vi "startTransport.vi"(8 "error in (no error)":errorcluster, 10 "method":T1, 11 "Inst.Transport in":refnum<class "Inst.Transport.lvclass">) -> (0 "error out":errorcluster, 3 "Inst.Transport out":refnum<class "Inst.Transport.lvclass">)   [LabVIEW 2019, in "Inst.Transport.lvclass"]
uses:
  Inst.Transport.lvclass
  Typedefs/Inst.Transport.PublicCommands--Enum.ctl
  Typedefs/startTransport--Request--Cluster.ctl
  Transport/Typedefs/Transport.Methods--Enum.ctl
  Transport/Transport.lvclass
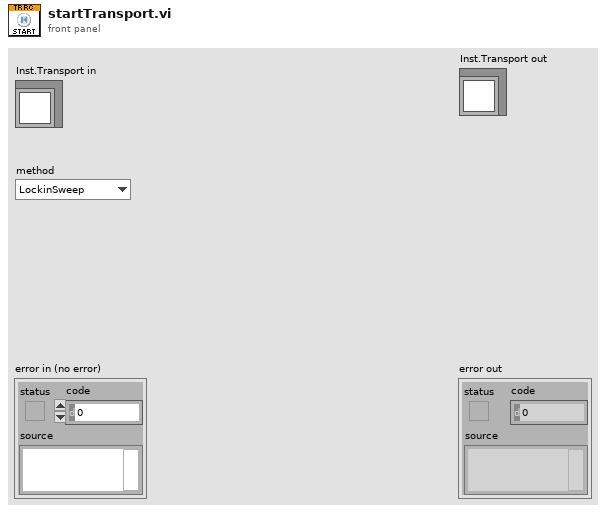
[diagram p1: front panel]
types:
  T1 = typedef "Transport.lvclass/Transport.Methods--Enum.ctl" = enum16{"LockinSweep", "LockinTime", "LockinTimeDelay"}
  T2 = typedef "Inst.Transport.lvclass/startTransport--Request--Cluster.ctl" = cluster{"method":T1}
  T3 = typedef "Inst.Transport.lvclass/Inst.Transport.PublicCommands--Enum.ctl" = enum16{"startTransport", "stopTransport", "getStatus", "setExptFolder", "getExptFolder", "setExptComments", "getExptComments", "setExptParam", "appendExptParam", "clearExptParam", "setSweepConfig", "getSweepConfig", "setRefreshTime"}
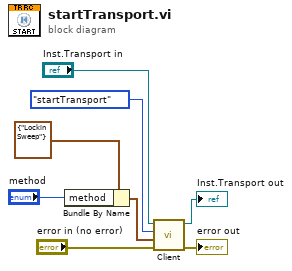
[diagram p0: block diagram]
diagram:
  n1 = Bundle By Name(cluster=T2 {"method"=enum."LockinSweep"} ("startTransport"), "method"="method") -> (w2:T2)
  n2 = call-dynamic "Client.vi"("error in (no error)"="error in (no error)", "Data in"=w2, "Command in"=Inst.Transport.PublicCommands--Enum."startTransport" ("Commands"), "Instrument in"="Inst.Transport in") -> ("error out"=→"error out":errorcluster, "Instrument out"=→"Inst.Transport out":refnum<class "Inst.Transport.lvclass">)  [unwired: 4 in, 2 out]
